vi "3 Balls.vi"(10 "Where":string) -> ()   [LabVIEW 2019]
uses:
  MotorsGlobal.vi
  JoysticksGlobal.vi
  TurretMode.ctl
  StateMachine_3BallLoadingBay.ctl
panel:
  in  "PIDs":T1(tab)
  in  "Anda1_TimeLimit":dbl
  in  "Distance1":dbl
  in  "DelayAnda1":i32=300
  in  "Setpoint_CurvaEsq1":dbl
  in  "GainsCurvaEsq1":T2={"proportional gain (Kc)"=1.0, "integral time (Ti, min)"=0.01, "derivative time (Td, min)"=0.0} {"derivative time (Td, min)" format="%.3f"; "integral time (Ti, min)" format="%.3f"; "proportional gain (Kc)" format="%.3f"}
  in  "RangeCurvaEsq1":cluster{"output high":dbl, "output low":dbl}={"output high"=0.6, "output low"=-0.6} {"output low" format="%.2f"; "output high" format="%.2f"}
  in  "CurvaEsq1_TimeLimit":dbl
  in  "Distance2":dbl
  in  "Anda2_TimeLimit":dbl
  in  "DelayAnda2":i32=300
  in  "GainsCurvaEsq2":T2={"proportional gain (Kc)"=1.0, "integral time (Ti, min)"=0.01, "derivative time (Td, min)"=0.0} {"derivative time (Td, min)" format="%.3f"; "integral time (Ti, min)" format="%.3f"; "proportional gain (Kc)" format="%.3f"}
  in  "RangeCurvaEsq2":cluster{"output high":dbl, "output low":dbl}={"output high"=0.6, "output low"=-0.6} {"output low" format="%.2f"; "output high" format="%.2f"}
  in  "Setpoint_CurvaEsq2":dbl
  in  "CurvaEsq2_TimeLimit":dbl
  in  "AlinhaLL_TimeLimit":dbl
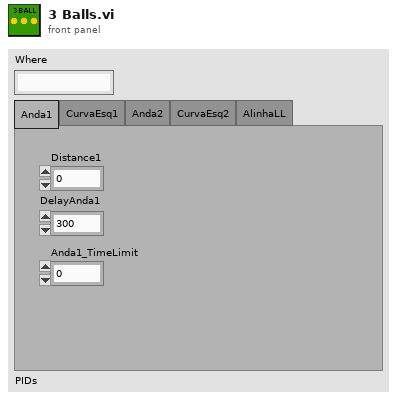
[diagram p1: front panel]
types:
  T1 = enum32{"Anda1", "CurvaEsq1", "Anda2", "CurvaEsq2", "AlinhaLL"}
  T2 = cluster{"proportional gain (Kc)":dbl, "integral time (Ti, min)":dbl, "derivative time (Td, min)":dbl}
  T3 = typedef "TurretMode.ctl" = enum16{"Static", "Manual", "Automatic"}
  T4 = typedef "StateMachine_3BallLoadingBay.ctl" = enum16{"Standart", "Anda1", "CurvaEsq1", "Reset1", "Anda2", "CurvaEsq2", "AlinhaLL", "Atira"}
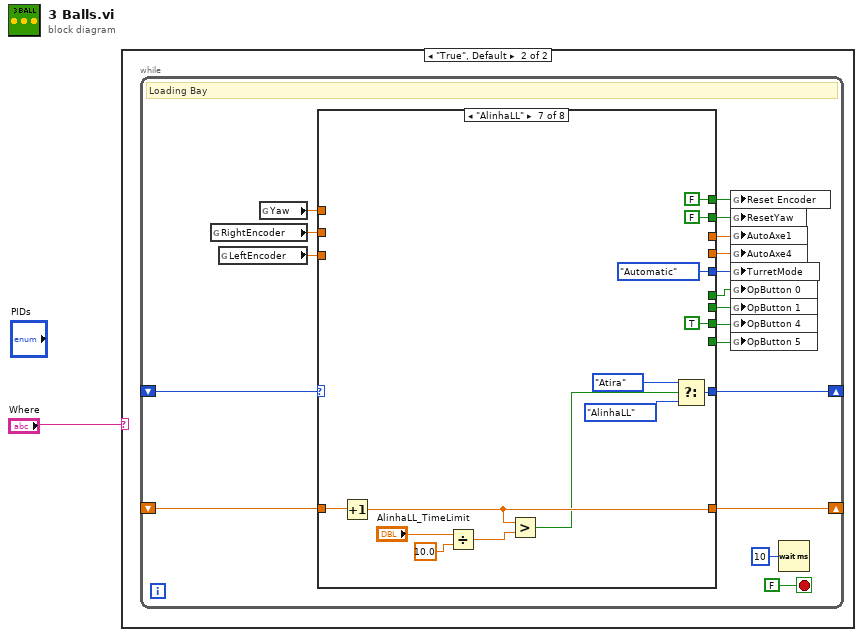
[diagram p0: block diagram]
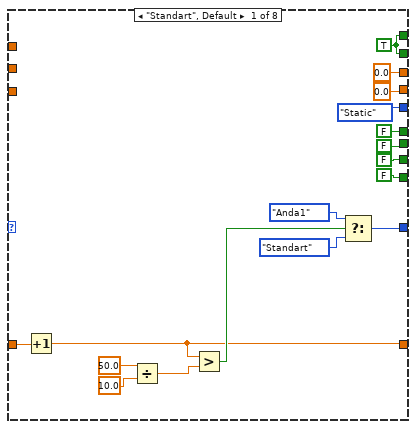
[diagram p3: hidden frame]
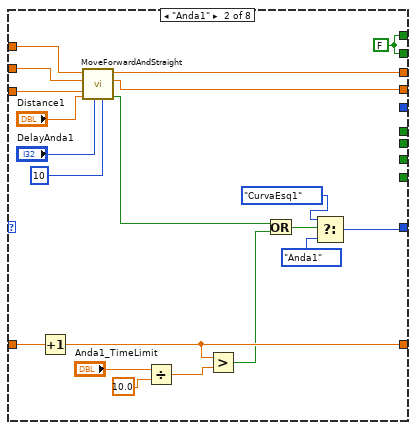
[diagram p4: hidden frame]
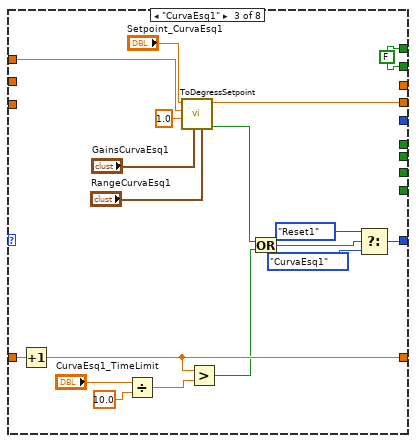
[diagram p5: hidden frame]
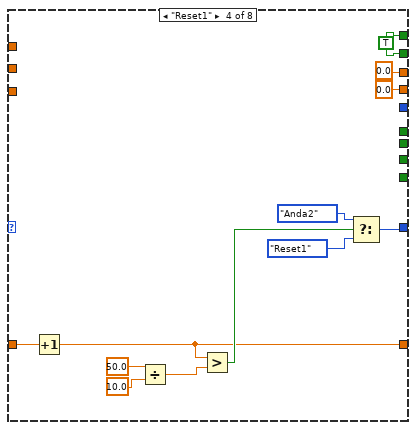
[diagram p6: hidden frame]
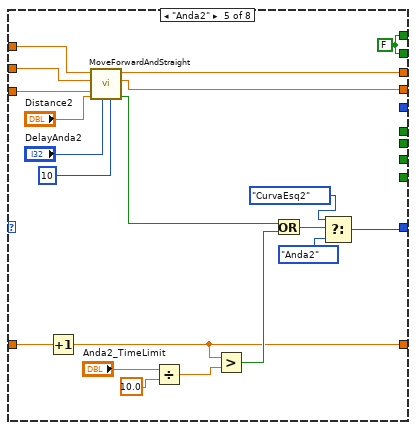
[diagram p7: hidden frame]
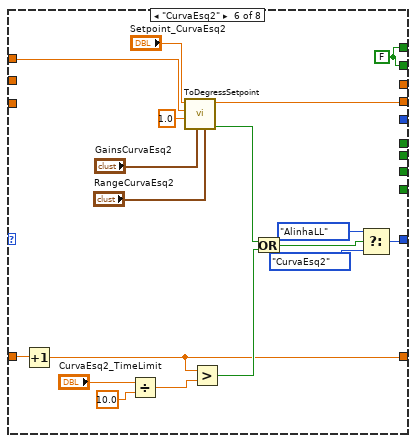
[diagram p8: hidden frame]
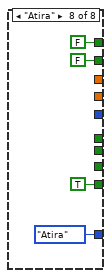
[diagram p9: hidden frame]
diagram:
  n1 = case shown="\"True\", Default" "Where" {
    frame "False" {
    }
    frame "True", Default {
      n2 = while {
        shift-right: [w7] -> _
        shift-left: _ -> [w19]
        shift-right: [w14] -> _
        shift-left: _ -> [w15]
        stop <- FALSE stop-if-true
        # "Loading Bay"
        n3 = global read "MotorsGlobal.vi" "RightEncoder"() -> (w17:dbl)
        n4 = global read "MotorsGlobal.vi" "LeftEncoder"() -> (w18:dbl)
        n5 = global read "MotorsGlobal.vi" "Yaw"() -> (w16:dbl)
        n6 = case shown="\"AlinhaLL\"" w19 {
          tunnel: w18 -> [_ w55 _ _ w93 _ _ _]
          tunnel: w17 -> [_ w54 _ _ w94 _ _ _]
          tunnel: w16 -> [_ w53 w74 _ w95 w109 _ _]
          tunnel: w15 -> [w31 w48 w65 w80 w92 w112 w133 _]
          tunnel: [w25 w46 w64 w79 w91 w111 w132 _] -> w14
          tunnel: [0.0 ("Direction") w40 w71 0.0 ("Direction") w90 w110 _ _] -> w11
          tunnel: [0.0 ("Trottle") w39 _ 0.0 ("Trottle") w89 _ _ _] -> w10
          tunnel: [w34 w38 w58 w78 w88 w108 FALSE FALSE] -> w9
          tunnel: [w34 w38 w58 w78 w88 w108 FALSE FALSE] -> w8
          tunnel: [w28 w37 w57 w75 w87 w107 w128 StateMachine_3BallLoadingBay."Atira"] -> w7
          tunnel: [TurretMode."Static" ("TurretMode") _ _ _ _ _ TurretMode."Automatic" ("TurretMode") _] -> w6
          tunnel: [FALSE ("OpButton 4") _ _ _ _ _ TRUE ("OpButton 4") _] -> w5
          tunnel: [FALSE ("OpButton 5") _ _ _ _ _ _ TRUE ("OpButton 5")] -> w4
          tunnel: [FALSE ("OpButton 5") _ _ _ _ _ _ _] -> w3
          tunnel: [FALSE ("OpButton 4") _ _ _ _ _ _ _] -> w2
          frame "Standart", Default {
            w34 = TRUE
            n7 = Increment(x=w31) -> (x+1=w25:dbl)
            n8 = Divide(x=50.0, y=10.0) -> (x/y=w33:dbl)
            n9 = Greater?(x=w25, y=w33) -> (0:w26:bool)
            n10 = Select(t=StateMachine_3BallLoadingBay."Anda1", s=w26, f=StateMachine_3BallLoadingBay."Standart") -> (s? t:f=w28:T4)
          }
          frame "Anda1" {
            w38 = FALSE
            n11 = Increment(x=w48) -> (x+1=w46:dbl)
            n12 = call "MoveForwardAndStraight.vi"("Loop Timer"=10, "Time to stop"="DelayAnda1", "Distance"="Distance1", "Encoder Left"=w55, "Encoder Right"=w54, "Yaw"=w53) -> ("Finished distance"=w49:bool, "Direction"=w40:dbl, "Trottle"=w39:dbl)  [unwired: 2 in, 1 out]
            n13 = Divide(x="Anda1_TimeLimit", y=10.0) -> (x/y=w47:dbl)
            n14 = Greater?(x=w46, y=w47) -> (0:w45:bool)
            n15 = Or(x=w49, y=w45) -> (x .or. y?=w44:bool)
            n16 = Select(t=StateMachine_3BallLoadingBay."CurvaEsq1", s=w44, f=StateMachine_3BallLoadingBay."Anda1") -> (s? t:f=w37:T4)
          }
          frame "CurvaEsq1" {
            w58 = FALSE
            n17 = Increment(x=w65) -> (x+1=w64:dbl)
            n18 = Divide(x="CurvaEsq1_TimeLimit", y=10.0) -> (x/y=w67:dbl)
            n19 = call "ToDegressSetpoint.vi"("Range"="RangeCurvaEsq1", "Gains"="GainsCurvaEsq1", "Precision"=1.0, "Yaw"=w74, "Setpoint (degress)"="Setpoint_CurvaEsq1") -> ("Finished?"=w59:bool, "Output"=w71:dbl)  [unwired: 5 in]
            n20 = Greater?(x=w64, y=w67) -> (0:w60:bool)
            n21 = Or(x=w59, y=w60) -> (x .or. y?=w61:bool)
            n22 = Select(t=StateMachine_3BallLoadingBay."Reset1", s=w61, f=StateMachine_3BallLoadingBay."CurvaEsq1") -> (s? t:f=w57:T4)
          }
          frame "Reset1" {
            w78 = TRUE
            n23 = Increment(x=w80) -> (x+1=w79:dbl)
            n24 = Divide(x=50.0, y=10.0) -> (x/y=w86:dbl)
            n25 = Greater?(x=w79, y=w86) -> (0:w81:bool)
            n26 = Select(t=StateMachine_3BallLoadingBay."Anda2", s=w81, f=StateMachine_3BallLoadingBay."Reset1") -> (s? t:f=w75:T4)
          }
          frame "Anda2" {
            w88 = FALSE
            n27 = Increment(x=w92) -> (x+1=w91:dbl)
            n28 = call "MoveForwardAndStraight.vi"("Loop Timer"=10, "Time to stop"="DelayAnda2", "Distance"="Distance2", "Encoder Left"=w93, "Encoder Right"=w94, "Yaw"=w95) -> ("Finished distance"=w102:bool, "Direction"=w90:dbl, "Trottle"=w89:dbl)  [unwired: 2 in, 1 out]
            n29 = Divide(x="Anda2_TimeLimit", y=10.0) -> (x/y=w101:dbl)
            n30 = Greater?(x=w91, y=w101) -> (0:w100:bool)
            n31 = Or(x=w102, y=w100) -> (x .or. y?=w99:bool)
            n32 = Select(t=StateMachine_3BallLoadingBay."CurvaEsq2", s=w99, f=StateMachine_3BallLoadingBay."Anda2") -> (s? t:f=w87:T4)
          }
          frame "CurvaEsq2" {
            w108 = FALSE
            n33 = Increment(x=w112) -> (x+1=w111:dbl)
            n34 = Divide(x="CurvaEsq2_TimeLimit", y=10.0) -> (x/y=w119:dbl)
            n35 = call "ToDegressSetpoint.vi"("Range"="RangeCurvaEsq2", "Gains"="GainsCurvaEsq2", "Precision"=1.0, "Yaw"=w109, "Setpoint (degress)"="Setpoint_CurvaEsq2") -> ("Finished?"=w113:bool, "Output"=w110:dbl)  [unwired: 5 in]
            n36 = Greater?(x=w111, y=w119) -> (0:w114:bool)
            n37 = Or(x=w113, y=w114) -> (x .or. y?=w115:bool)
            n38 = Select(t=StateMachine_3BallLoadingBay."AlinhaLL", s=w115, f=StateMachine_3BallLoadingBay."CurvaEsq2") -> (s? t:f=w107:T4)
          }
          frame "AlinhaLL" {
            n39 = Increment(x=w133) -> (x+1=w132:dbl)
            n40 = Divide(x="AlinhaLL_TimeLimit", y=10.0) -> (x/y=w135:dbl)
            n41 = Greater?(x=w132, y=w135) -> (0:w129:bool)
            n42 = Select(t=StateMachine_3BallLoadingBay."Atira", s=w129, f=StateMachine_3BallLoadingBay."AlinhaLL") -> (s? t:f=w128:T4)
          }
          frame "Atira" {
          }
        }
        n43 = global write "MotorsGlobal.vi" "Reset Encoder"(w9) -> ()
        n44 = global write "MotorsGlobal.vi" "ResetYaw"(w8) -> ()
        n45 = global write "JoysticksGlobal.vi" "AutoAxe1"(w10) -> ()
        n46 = global write "JoysticksGlobal.vi" "AutoAxe4"(w11) -> ()
        n47 = global write "MotorsGlobal.vi" "TurretMode"(w6) -> ()
        n48 = global write "JoysticksGlobal.vi" "OpButton 0"(w2) -> ()
        n49 = global write "JoysticksGlobal.vi" "OpButton 1"(w3) -> ()
        n50 = global write "JoysticksGlobal.vi" "OpButton 4"(w5) -> ()
        n51 = global write "JoysticksGlobal.vi" "OpButton 5"(w4) -> ()
        n52 = Wait (ms)(milliseconds to wait=u32 10) -> ()  [unwired: 1 out]
      }
    }
  }
